vi "Get Monkey Sync Flag.vi"(8 "error in (no error)":errorcluster, 10 "Monkey ID":string, 11 "Tamer in":refnum<class "Tamer.lvclass">=refnum) -> (0 "error out":errorcluster, 2 "Monkey Sync Flag":bool, 3 "Tamer out":refnum<class "Tamer.lvclass">)   [LabVIEW 2020, in "CIRCUS_uServices.lvlib" / "Holy Trinity.lvlib" / "Tamer.lvlib" / "Tamer.lvclass"]
uses:
  Tamer.lvclass
  TALOS/TALOS_PPL.lvlibp
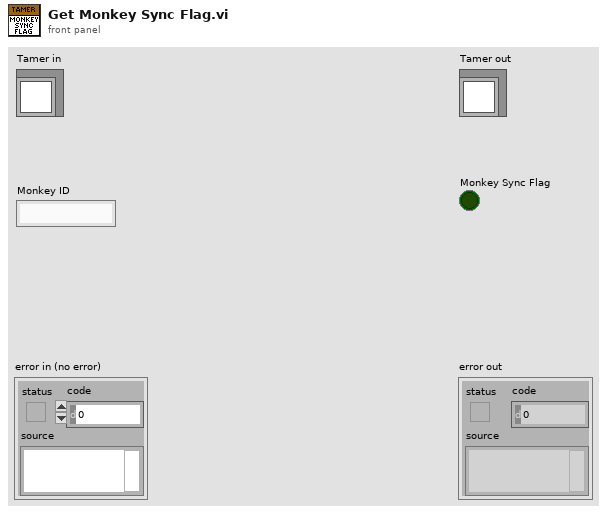
[diagram p1: front panel]
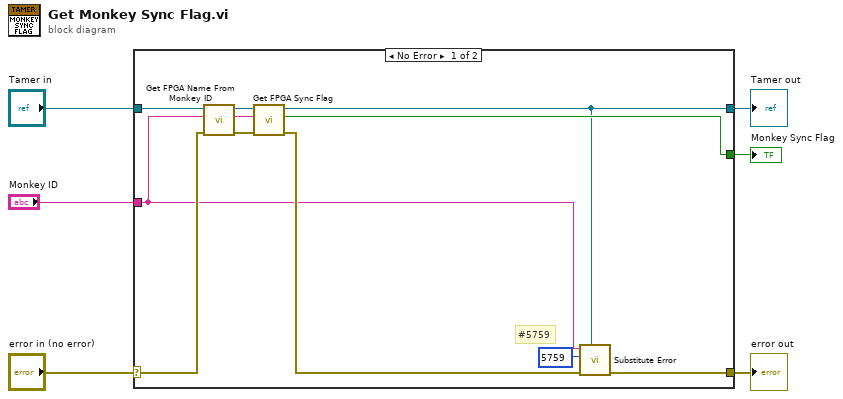
[diagram p0: block diagram]
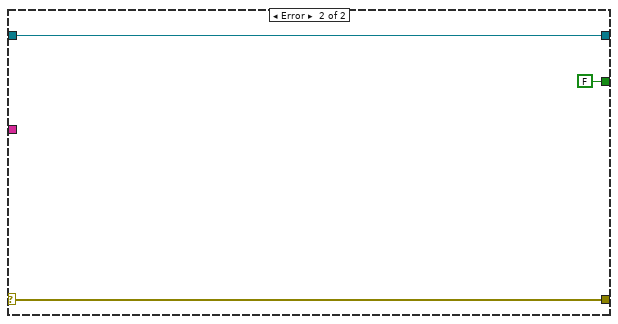
[diagram p2: hidden frame]
diagram:
  n1 = case shown="No Error" "error in (no error)" {
    selector: "error in (no error)" -> [w16 w20]
    tunnel: [w9 w20] -> w5
    tunnel: [w8 w19] -> w3
    tunnel: "Tamer in" -> [w17 w19]
    tunnel: "Monkey ID" -> [w7 _]
    tunnel: [w12 FALSE ("f")] -> w1
    frame No Error {
      # "#5759"
      n2 = call-dynamic "Get FPGA Name From Monkey ID.vi"("error in (no error)"=w16, "Monkey ID"=w7, "Tamer in"=w17) -> ("error out"=w13:errorcluster, "FPGA Name"=w14:string, "Tamer out"=w15:refnum<class "Tamer.lvclass">)  [unwired: 6 in]
      n3 = call-dynamic "Get FPGA Sync Flag.vi"("error in (no error)"=w13, "FPGA Name"=w14, "Tamer in"=w15) -> ("error out"=w10:errorcluster, "FPGA Sync Flag"=w12:bool, "Tamer out"=w8:refnum<class "Tamer.lvclass">)  [unwired: 6 in]
      n4 = call "Substitute Error.vi"("LabVIEW Object"=w8, "error in (no error)"=w10, "Error Code"=5759, "Optional String"=w7) -> ("error out"=w9:errorcluster)  [unwired: 7 in]
    }
    frame Error {
    }
  }
  "error out" <- w5
  "Tamer out" <- w3
  "Monkey Sync Flag" <- w1
